vi "VI Tree.vi"   [LabVIEW 2017, in "BK Precision 1823A.lvlib"]
doc: "This is the instrument driver for the B&K Precision 1823A frequency counter. The VI Tree displays all the user-callable VIs of the instrument driver in an organized table."
uses:
  <instrlib>/BK Precision 1823A/BK Precision 1823A.lvlib
panel:
  # "(c) 2009 B&K PRECISION CORPORATION.  ALL RIGHTS RESERVED."
  # "SEE DIAGRAM\nFOR VI TREE."
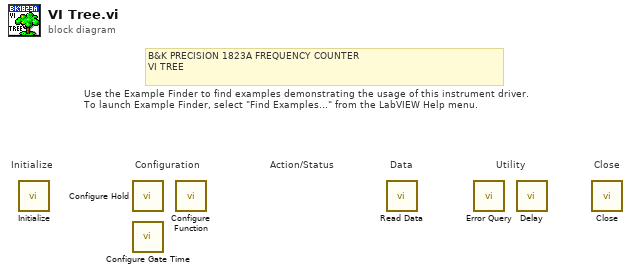
[diagram p0: block diagram]
diagram:
  # "B&K PRECISION 1823A FREQUENCY COUNTER\nVI TREE"
  # "Use the Example Finder to find examples demonstrating the usage of this instrument driver.\nTo launch Example Finder, select \"Find Examples...\" from the LabVIEW Help menu."
  # "Configuration"
  # "Utility"
  # "Data"
  # "Action/Status"
  # "Close"
  # "Initialize"
  n1 = call <instrlib>:"Initialize.vi"() -> ()  [unwired: 10 in, 2 out]
  n2 = call <instrlib>:"Configure Hold.vi"() -> ()  [unwired: 10 in, 2 out]
  n3 = call <instrlib>:"Configure Gate Time.vi"() -> ()  [unwired: 10 in, 2 out]
  n4 = call <instrlib>:"Configure Function.vi"() -> ()  [unwired: 10 in, 2 out]
  n5 = call <instrlib>:"Read Data.vi"() -> ()  [unwired: 8 in, 4 out]
  n6 = call <instrlib>:"Error Query.vi"() -> ()  [unwired: 10 in, 2 out]
  n7 = call <instrlib>:"Delay.vi"() -> ()  [unwired: 10 in, 2 out]
  n8 = call <instrlib>:"Close.vi"() -> ()  [unwired: 11 in, 1 out]
